vi "temp.vi"() -> ()   [LabVIEW 2020, in "C-887.lvclass"]
uses:
  C-887.lvclass
  LabVIEW/Low Level/Communication.llb/Interface Settings.ctl
panel:
  in  "PI Interface settings":T1={"Interface"=4, "Timeout"=5000, "RS232 settings"={"Portnumber"=1, "Baudrate"=5}, "TCP/IP settings"={"Host address/name"="localhost", "Port"=50000, "Board"=0, "TCP/IP Search?"=TRUE}, "USB settings"={"S/N"="", "USB Search?"=TRUE}, "DaisyChain settings"={"Register DC"=FALSE, "DaisyChain Search?"=TRUE, "Device ID"=1}, "DLL for Device"=0} {"DLL for Device" items=["None", "C-843", "C-844", "E-710", "C-843.PM", "C-865", "E-761", "Mercury", "E-755", "E-753", "C-866", "E-712", "E-725", "E-861", "C-867", "E-517", "E-816", "E-709", "PI_GCS2_DLL", "HydraPollux"]; "Interface" items=["RS232", "RS232 DaisyChain", "USB", "USB DaisyChain", "TCP/IP", "TCP/IP DaisyChain", "PCI"]; "RS232 settings"."Portnumber" min=1 step=1; "RS232 settings"."Baudrate" items=["9600", "14400", "19200", "38400", "57600", "115200", "230400", "460800"]}
  in  "error in (no error)":errorcluster
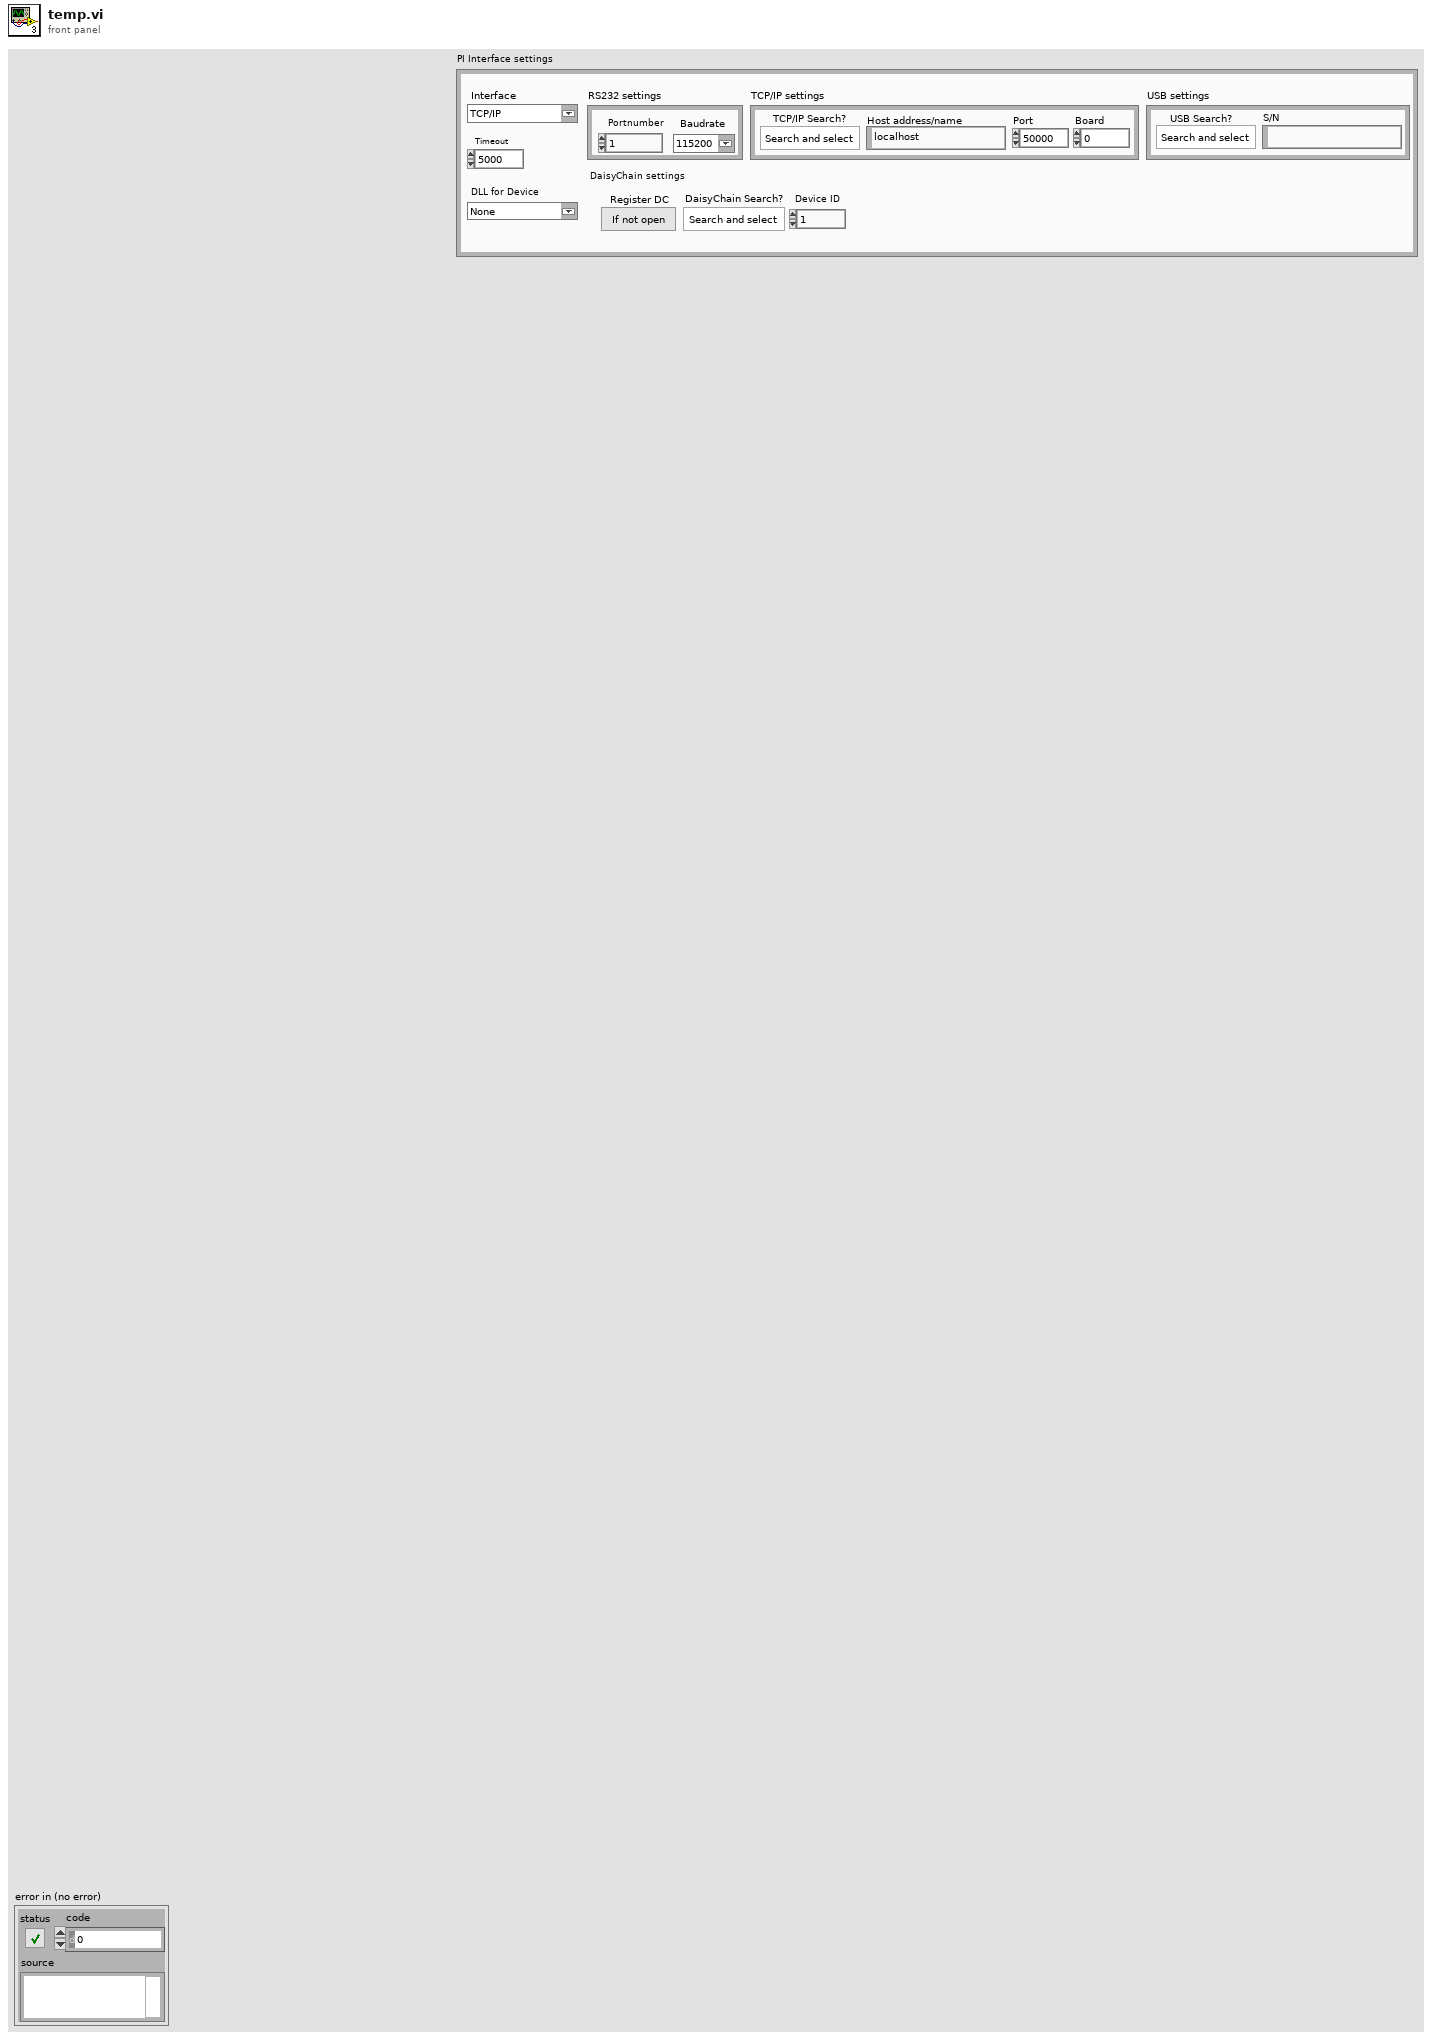
[diagram p1: front panel]
types:
  T1 = typedef "Interface Settings.ctl" = cluster{"Interface":u16, "Timeout":u32, "RS232 settings":cluster{"Portnumber":u8, "Baudrate":u16}, "TCP/IP settings":cluster{"Host address/name":string, "Port":i32, "Board":i32, "TCP/IP Search?":bool}, "USB settings":cluster{"S/N":string, "USB Search?":bool}, "DaisyChain settings":cluster{"Register DC":bool, "DaisyChain Search?":bool, "Device ID":i32}, "DLL for Device":u16}
  T2 = typedef "HexapodPI.lvclass/settingHexapod_TypDEf.ctl" = cluster{"xpos":cluster{"Value":dbl, "Min":dbl, "Max":dbl, "StepSize":dbl, "Tolerance":dbl, "ValueActual":dbl}, "ypos":cluster{"Value":dbl, "Min":dbl, "Max":dbl, "StepSize":dbl, "Tolerance":dbl, "ValueActual":dbl}, "zpos":cluster{"Value":dbl, "Min":dbl, "Max":dbl, "StepSize":dbl, "Tolerance":dbl, "ValueActual":dbl}, "uangle":cluster{"Value":dbl, "Min":dbl, "Max":dbl, "StepSize":dbl, "Tolerance":dbl, "ValueActual":dbl}, "vangle":cluster{"Value":dbl, "Min":dbl, "Max":dbl, "StepSize":dbl, "Tolerance":dbl, "ValueActual":dbl}, "devaddress":string, "connectiontype":enum16{"TCPIP", "Serial"}, "hexinit":enum16{"Not referenced", "Referenced"}, "status":enum16{"Not referenced", "Homing", "Moving", "Ready"}, "relativeMove":cluster{"Zpos":T3, "Zneg":T3, "Xpos":T3, "Xneg":T3, "Ypos":T3, "Yneg":T3, "Wpos":T3, "Wneg":T3, "Vpos":T3, "Vneg":T3, "Upos":T3, "Uneg":T3}, "stepsize":cluster{"Value":dbl, "Min":dbl, "Max":dbl, "StepSize":dbl, "Tolerance":dbl, "ValueActual":dbl}, "LaserAxis":cluster{"u":dbl, "v":dbl, "w":dbl}, "PivotPoint":T4, "wangle":cluster{"Value":dbl, "Min":dbl, "Max":dbl, "StepSize":dbl, "Tolerance":dbl, "ValueActual":dbl}, "LaserAxes":T3, "speed":cluster{"Value":dbl, "Min":dbl, "Max":dbl, "StepSize":dbl, "Tolerance":dbl, "ValueActual":dbl}, "Simulation":T3, "xyzuvw":dbl[], "xyzuvw_tolerances":dbl[]}
  T3 = typedef "OnOffTypeDef.ctl" = enum16{"off", "on"}
  T4 = typedef "PivotPoint_TypDef.ctl" = cluster{"R":cluster{"Value":dbl, "Min":dbl, "Max":dbl, "StepSize":dbl, "Tolerance":dbl, "ValueActual":dbl}, "S":cluster{"Value":dbl, "Min":dbl, "Max":dbl, "StepSize":dbl, "Tolerance":dbl, "ValueActual":dbl}, "T":cluster{"Value":dbl, "Min":dbl, "Max":dbl, "StepSize":dbl, "Tolerance":dbl, "ValueActual":dbl}}
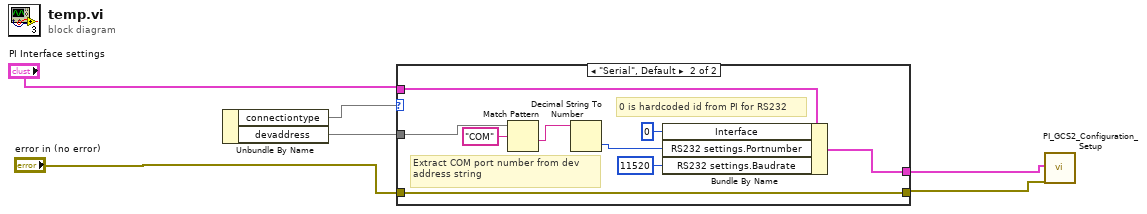
[diagram p0: block diagram]
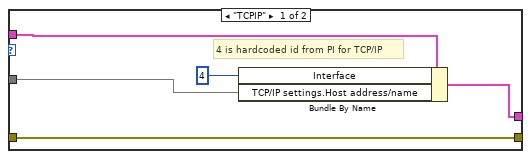
[diagram p2: hidden frame]
diagram:
  n1 = Unbundle By Name() -> (w7:T2, "connectiontype"=w6, "devaddress"=w1)
  n2 = case shown="\"Serial\", Default" w6 {
    tunnel: "error in (no error)" -> [w12 w18]
    tunnel: "PI Interface settings" -> [w10 w21]
    tunnel: [w11 w20] -> w3
    tunnel: [w12 w18] -> w2
    tunnel: w1 -> [w8 w16]
    frame "TCPIP" {
      # "4 is hardcoded id from PI for TCP/IP"
      n3 = Bundle By Name(cluster=w10, "Interface"=u16 4, "TCP/IP settings.Host address/name"=w8) -> (w11:T1)
    }
    frame "Serial", Default {
      # "0 is hardcoded id from PI for RS232"
      # "Extract COM port number from dev address string"
      n4 = Match Pattern(string=w16, regular expression="COM") -> (after substring=w14:string)  [unwired: 1 in, 3 out]
      n5 = Decimal String To Number(string=w14) -> (number=w13:i32)  [unwired: 2 in, 1 out]
      n6 = Bundle By Name(cluster=w21, "Interface"=u16 0, "RS232 settings.Portnumber"=w13, "RS232 settings.Baudrate"=u16 11520) -> (w20:T1)
    }
  }
  n7 = call "PI_GCS2_Configuration_Setup.vi"("Interface settings"=w3, "error in"=w2) -> ()  [unwired: 12 in, 6 out]
